vi "Simple Filter Print to Serial.vi"(8 "error in":errorcluster) -> (0 "error out":errorcluster)   [LabVIEW 2014]
doc: "DEMO 423 - Digital Filter for Arduino\n\nSimple shows how to implement filter in diagram and after rewrite it into arduino code. This filter is also able to run on desktop application for testing."
uses:
  <vilib>/LabVIEW Universal Transcriptor/LabVIEW to Arduino Transcriptor/Transcriptors/System API/Serial println string.vi
  <vilib>/LabVIEW Universal Transcriptor/LabVIEW to Arduino Transcriptor/Transcriptors/System API/Serial print string.vi
  <vilib>/LabVIEW Universal Transcriptor/LabVIEW for Arduino Math Library/Arduino Math.lvlib
  <vilib>/LabVIEW Universal Transcriptor/LabVIEW to Arduino Transcriptor/Transcriptors/System API/System Serial Library Variables/System Serial Library Variables.lvlib
panel:
  out "String Buffer":string=" "
  out "signal in":sgl[](graph)
  in  "signal type":u16(ring) items=["sine", "user"]
  out "signal out":sgl[](graph)
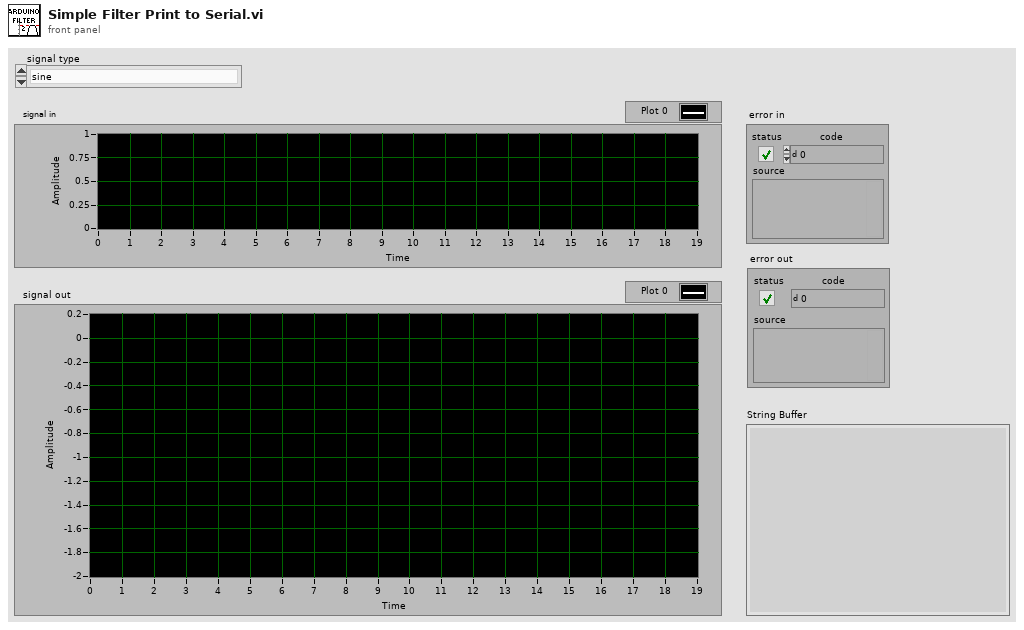
[diagram p1: front panel]
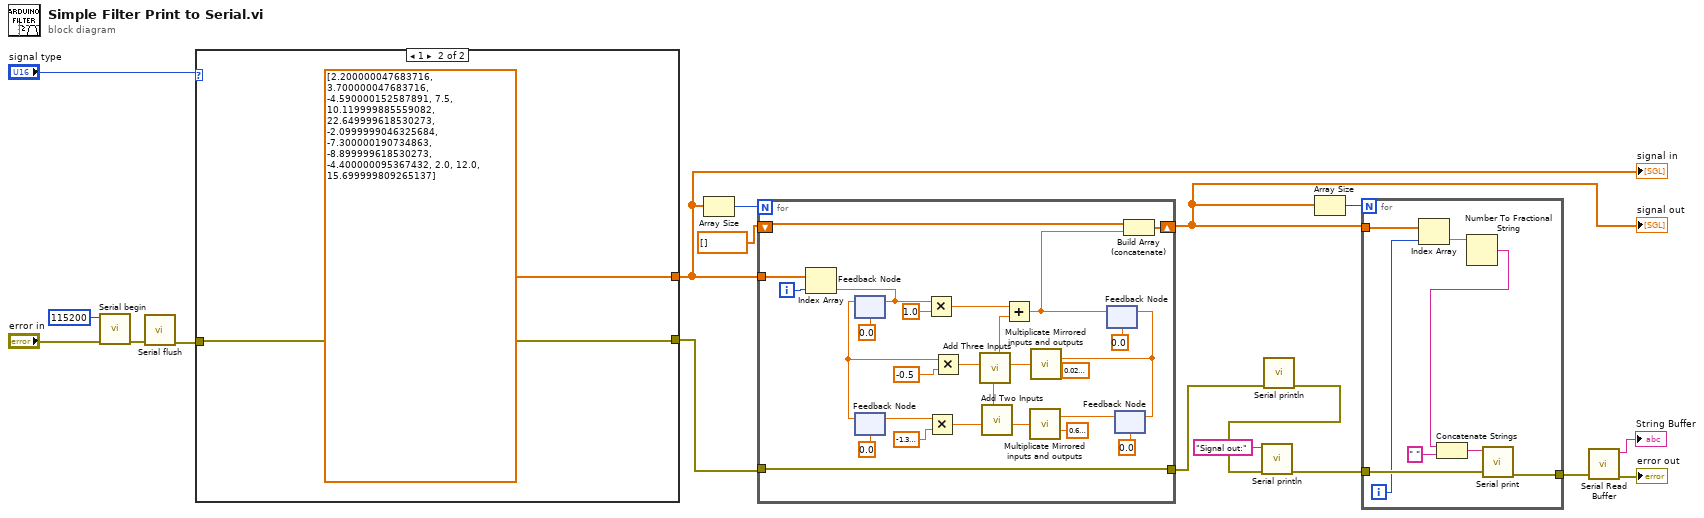
[diagram p0: block diagram]
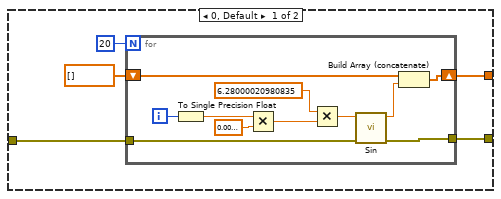
[diagram p2: hidden frame]
diagram:
  n1 = call <vilib>:"Serial begin.vi"("Error In"="error in", "speed (Bd)"=115200) -> ("Error Out"=w4:errorcluster)  [unwired: 9 in]
  n2 = call <vilib>:"Serial flush.vi"("Error In"=w4) -> ("Error Out"=w3:errorcluster)  [unwired: 10 in]
  n3 = case shown="1" "signal type" {
    tunnel: [w20 sgl[] [2.2, 3.7, -4.59, 7.5, 10.12, 22.65, -2.1, -7.3, -8.9, -4.4, 2.0, 12.0, 15.7]] -> w15
    tunnel: w3 -> [w22 w35]
    tunnel: [w19 w35] -> w14
    frame 0, Default {
      n4 = for {
        N: 20 -> [_]
        tunnel: w22 -> [w34]
        shift-right: [w27] -> w20
        shift-left: sgl[] [] -> [w25]
        tunnel: [w24] -> w19
        i -> [w32]
        n5 = To Single Precision Float(number=w32) -> (single precision float=w30:sgl)
        n6 = Multiply(x=w30, y=sgl 0.01) -> (x*y=w29:sgl)
        n7 = Multiply(x=sgl 6.28, y=w29) -> (x*y=w28:sgl)
        n8 = call <vilib>:"Sin.vi"("Error In"=w34, "x"=w28) -> ("Error Out"=w24:errorcluster, "sin(x)"=w26:sgl)  [unwired: 8 in]
        n9 = Build Array (concatenate)(w25, w26) -> (w27:sgl[])
      }
    }
    frame 1 {
    }
  }
  "signal in" <- w15
  n10 = Array Size(array=w15) -> (size(s)=w18:i32)
  n11 = for {
    N: w18 -> [_]
    tunnel: w15 -> [w63]
    shift-right: [w61] -> w8
    shift-left: sgl[] [] -> [w60]
    tunnel: [w37] -> w2
    tunnel: w14 -> [w37]
    i -> [w62]
    n12 = Index Array(array=w63, index=w62) -> (element=w53:sgl)
    n13 = feedback #1(sgl 0.0 ("sin(x)")) -> (w48:sgl)
    n14 = feedback-in #1(w53) -> ()
    n15 = feedback #2(sgl 0.0 ("sin(x)")) -> (w45:sgl)
    n16 = feedback-in #2(w48) -> ()
    n17 = Multiply(x=w53, y=sgl 1.0) -> (x*y=w52:sgl)
    n18 = Multiply(x=w45, y=sgl -1.4) -> (x*y=w46:sgl)
    n19 = Multiply(x=w48, y=sgl -0.5) -> (x*y=w49:sgl)
    n20 = feedback #3(sgl 0.0 ("sin(x)")) -> (w42:sgl)
    n21 = call "Multiplicate Mirrored inputs and outputs.vi"("in 1"=w42, "in 2"=sgl 0.03) -> ("out"=w43:sgl)  [unwired: 13 in]
    n22 = feedback #4(sgl 0.0 ("sin(x)")) -> (w39:sgl)
    n23 = call "Multiplicate Mirrored inputs and outputs.vi"("in 1"=w39, "in 2"=sgl 0.7) -> ("out"=w38:sgl)  [unwired: 13 in]
    n24 = call "Add Two Inputs.vi"("in 2"=w38, "in 1"=w46) -> ("Numeric"=w54:sgl)  [unwired: 9 in]
    n25 = call "Add Three Inputs.vi"("in 2"=w43, "in 3"=w54, "in 1"=w49) -> ("Numeric"=w55:sgl)  [unwired: 8 in]
    n26 = Add(x=w52, y=w55) -> (x+y=w44:sgl)
    n27 = feedback-in #3(w44) -> ()
    n28 = feedback-in #4(w42) -> ()
    n29 = Build Array (concatenate)(w60, w44) -> (w61:sgl[])
  }
  "signal out" <- w8
  n30 = call-poly <vilib>:"Serial println.vi"("Error In"=w2) -> ("Error Out"=w1:errorcluster)  [unwired: 10 in]
  n31 = call-poly <vilib>:"Serial println.vi"("Error In"=w1, "string in"="Signal out:") -> ("Error Out"=w10:errorcluster)  [unwired: 9 in]
  n32 = Array Size(array=w8) -> (size(s)=w9:i32)
  n33 = for {
    N: w9 -> [_]
    tunnel: w10 -> [w71]
    tunnel: w8 -> [w68]
    tunnel: [w64] -> w7
    i -> [w67]
    n34 = Index Array(array=w68, index=w67) -> (element=w66:sgl)
    n35 = Number To Fractional String(number=w66) -> (F-format string=w65:string)  [unwired: 3 in]
    n36 = Concatenate Strings(w65, " " ("string")) -> (w70:string)
    n37 = call-poly <vilib>:"Serial print.vi"("Error In"=w71, "string in"=w70) -> ("Error Out"=w64:errorcluster)  [unwired: 9 in]
  }
  n38 = call <vilib>:"Serial Read Buffer.vi"("Error In"=w7) -> ("Error Out"=→"error out":errorcluster, "String Buffer"=→"String Buffer":string)  [unwired: 9 in]
